vi "Write Bitfile exe dir.vi"(8 "error in (no error)":errorcluster, 10 "Bitfile exe dir":path, 11 "io configuration in":refnum<class "io configuration.lvclass">) -> (0 "error out":errorcluster, 3 "io configuration out":refnum<class "io configuration.lvclass">)   [LabVIEW 2017, in "io configuration.lvclass"]
uses:
  io configuration.lvclass
  io configuration.lvclass/io configuration.ctl
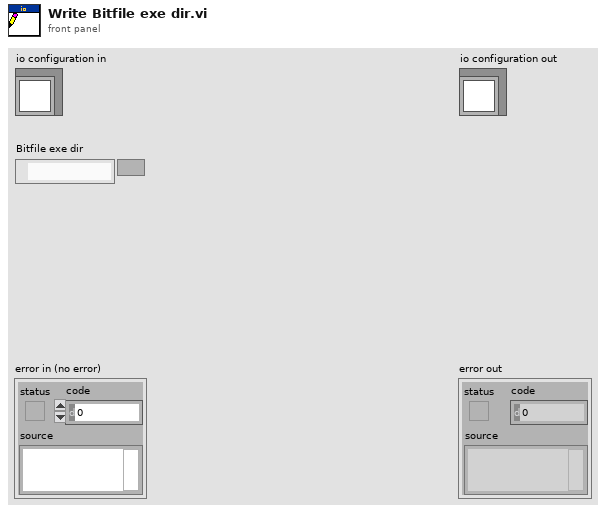
[diagram p1: front panel]
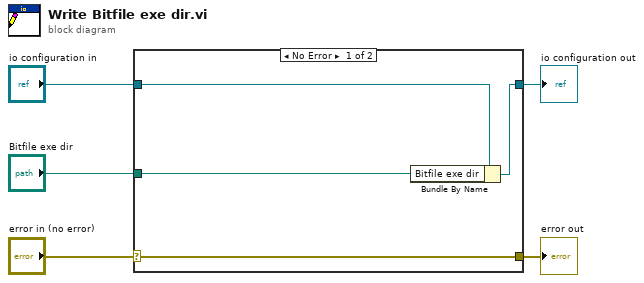
[diagram p0: block diagram]
diagram:
  n1 = case shown="No Error" "error in (no error)" {
    selector: "error in (no error)" -> [w9 w10]
    tunnel: [w9 w10] -> w4
    tunnel: [w7 w11] -> w2
    tunnel: "io configuration in" -> [w8 w11]
    tunnel: "Bitfile exe dir" -> [w6 _]
    frame No Error {
      n2 = Bundle By Name(cluster=w8, "Bitfile exe dir"=w6) -> (w7:refnum<class "io configuration.lvclass">)
    }
    frame Error {
    }
  }
  "error out" <- w4
  "io configuration out" <- w2
